vi "AIM664 Wait For Good Link.vi"(8 "error in":errorcluster, 10 "timeout (secs)":i32=10, 11 "InstrumentHandle_board in":u32) -> (0 "error out":errorcluster, 2 "Goodlink":bool, 3 "InstrumentHandle_board out":u32)   [LabVIEW 2020]
doc: "Check goodlink on port 0.\nTimeout 10 seconds if no goodlink established. Set custom error code -8110"
uses:
  typedefs/BoardControlIn.ctl
  typedefs/BoardControlGoodLink.ctl
  src/AIM664LV.lvlib
panel:
  in  "Board Control In":T1 {"Expert4Mode" items=["FDX_EXPERT_MODE", "FDX_DISA_GHOST"]; "Expert3Mode" items=["FDX_EXPERT_MODE", "FDX_DISA_GHOST"]; "Expert2Mode" items=["FDX_EXPERT_MODE", "FDX_DISA_GHOST"]; "Expert1Mode" items=["FDX_EXPERT_MODE", "FDX_DISA_GHOST"]; "Port4SpeedIn" items=["FDX_100MBIT", "FDX_10MBIT", "FDX_AUTO_100MBIT", "FDX_AUTO_10MBIT"]; "Port3SpeedIn" items=["FDX_100MBIT", "FDX_10MBIT", "FDX_AUTO_100MBIT", "FDX_AUTO_10MBIT"]; "Port2SpeedIn" items=["FDX_100MBIT", "FDX_10MBIT", "FDX_AUTO_100MBIT", "FDX_AUTO_10MBIT"]; "Port1SpeedIn" items=["FDX_100MBIT", "FDX_10MBIT", "FDX_AUTO_100MBIT", "FDX_AUTO_10MBIT"]; "Port4ConfigIn" items=["FDX_SINGLE", "FDX_REDUNDANT"]; "Port3ConfigIn" items=["FDX_SINGLE", "FDX_REDUNDANT"]; "Port2ConfigIn" items=["FDX_SINGLE", "FDX_REDUNDANT"]; "Port1ConfigIn" items=["FDX_SINGLE", "FDX_REDUNDANT"]; "Control" items=["FDX_READ", "FDX_WRITE"]}
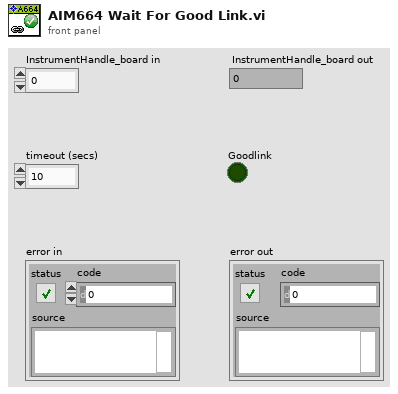
[diagram p1: front panel]
types:
  T1 = typedef "BoardControlIn.ctl" = cluster{"Control":u32, "Port1ConfigIn":u32, "Port2ConfigIn":u32, "Port3ConfigIn":u32, "Port4ConfigIn":i32, "Port1SpeedIn":u32, "Port2SpeedIn":u32, "Port3SpeedIn":u32, "Port4SpeedIn":u32, "Expert1Mode":u32, "Expert2Mode":u32, "Expert3Mode":u32, "Expert4Mode":u32, "RxVeriModeIn":u32, "RxVeriData1":u32, "RxVeriData2":u32, "RxVeriData3":u32, "RxVeriData4":u32, "RxVeriData5":u32, "RxVeriData6":u32, "RxVeriData7":u32, "RxVeriMask1":u32, "RxVeriMask2":u32, "RxVeriMask3":u32, "RxVeriMask4":u32, "RxVeriMask5":u32, "RxVeriMask6":u32, "RxVeriMask7":u32, "RxVerData8":u32, "RxVeriMask8":u32}
  T2 = typedef "BoardControlGoodLink.ctl" = u32
  T3 = cluster{"PortConfig":u32[], "PortSpeed":u32[], "PortUsed":u32[], "PortGoodLink":u32[], "ExpertMode":u32[], "GlobalMemFree":u32, "SharedMemFree":u32, "RxVeriMode":u32}
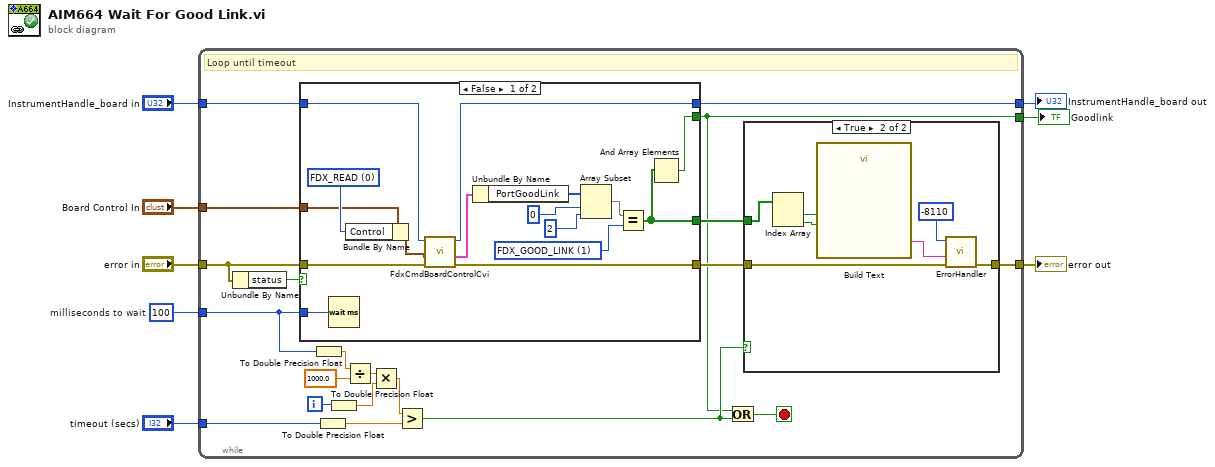
[diagram p0: block diagram]
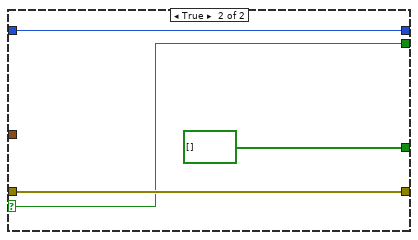
[diagram p2: hidden frame]
diagram:
  w3 = u32 100  # milliseconds to wait
  n1 = while {
    tunnel: "error in" -> [w28]
    tunnel: [w26] -> w7
    tunnel: "InstrumentHandle_board in" -> [w25]
    tunnel: "timeout (secs)" -> [w16]
    tunnel: [w12] -> w4
    tunnel: w3 -> [w11]
    tunnel: [w10] -> w2
    tunnel: "Board Control In" -> [w9]
    i -> [w20]
    stop <- w23 stop-if-true
    # "Loop until timeout"
    n2 = Unbundle By Name(w28) -> ("status"=w24:bool)
    n3 = case shown="False" w24 {
      selector: w24 -> [_ w47]
      tunnel: w25 -> [w42 w45]
      tunnel: w28 -> [w44 w48]
      tunnel: [w43 w48] -> w27
      tunnel: [w33 w47] -> w12
      tunnel: [w32 bool[] []] -> w21
      tunnel: w11 -> [w31 _]
      tunnel: [w30 w45] -> w10
      tunnel: w9 -> [w29 _]
      frame False {
        w38 = T2 1 items=["FDX_NO_LINK", "FDX_GOOD_LINK"] ("BoardControlGoodLink")
        w39 = u32 0 items=["FDX_READ", "FDX_WRITE"] ("Control")
        n4 = Wait (ms)(milliseconds to wait=w31) -> ()  [unwired: 1 out]
        n5 = Bundle By Name(cluster=w29, "Control"=w39) -> (w40:T1)
        n6 = call "FdxCmdBoardControlCvi.vi"("error in"=w44, "BoardControlIn (read)"=w40, "InstrumentHandle_board in"=w42) -> ("error out"=w43:errorcluster, "Board Control Out"=w41:T3, "InstrumentHandle_board out"=w30:u32)  [unwired: 6 in]
        n7 = Unbundle By Name(w41) -> ("PortGoodLink"=w37:u32[])
        n8 = Array Subset(array=w37, index=0, length=2) -> (w34:u32[])
        n9 = Equal?(x=w34, y=w38) -> (x = y?=w32:bool[])
        n10 = And Array Elements(Boolean array=w32) -> (logical AND=w33:bool)
      }
      frame True {
      }
    }
    n11 = To Double Precision Float(number=w11) -> (double precision float=w14:dbl)
    n12 = To Double Precision Float(number=w16) -> (double precision float=w18:dbl)
    n13 = To Double Precision Float(number=w20) -> (double precision float=w19:dbl)
    n14 = Divide(x=w14, y=1000.0) -> (x/y=w13:dbl)
    n15 = Multiply(x=w13, y=w19) -> (x*y=w17:dbl)
    n16 = Greater?(x=w17, y=w18) -> (0:w22:bool)
    n17 = Or(x=w12, y=w22) -> (x .or. y?=w23:bool)
    n18 = case shown="True" w22 {
      tunnel: w27 -> [w49 w56]
      tunnel: [w49 w55] -> w26
      tunnel: w21 -> [_ w54]
      frame False {
      }
      frame True {
        n19 = Index Array(array=w54) -> (element #1=w53:bool, element #2=w52:bool)  [unwired: 2 in]
        n20 = call "Build Text"("port1"=w53, "port2"=w52) -> ("Result"=w50:string)  [unwired: 12 in, 1 out]
        n21 = call "ErrorHandler.vi"("error in"=w56, "Custom Message"=w50, "AIM Error"=-8110 ("code")) -> ("error out"=w55:errorcluster)  [unwired: 8 in]
      }
    }
  }
  "error out" <- w7
  "Goodlink" <- w4
  "InstrumentHandle_board out" <- w2
